vi "Launch.vi"() -> ()   [LabVIEW 2013]
uses:
  Launchcontrol.ctl
panel:
  out "error out":errorcluster
  in  "error in (no error)":errorcluster
  in  "Engaged Angle":i32
  in  "Disengaged Angle":i32
  in  "A":bool
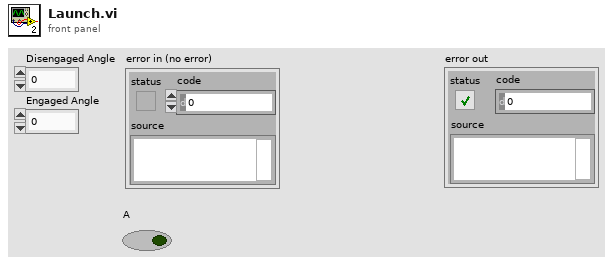
[diagram p1: front panel]
types:
  T1 = typedef "Launchcontrol.ctl" = enum16{"Engaging", "Waiting for Time to Elapse", "Disengaging", "Waiting for Button Press"}
  T2 = typedef "WPI_ServoDeviceRef.ctl" = cluster{"DeviceStatus":errorcluster, "Digital Module":T3, "PWM Channel":T4, "DeadBand":T5}
  T3 = typedef "FPGA_TypedefDigitalModule.ctl" = enum16{"Digital Module 1", "Digital Module 2"}
  T4 = typedef "FPGA_DIOPWMChannel.ctl" = enum8{"PWM 1", "PWM 2", "PWM 3", "PWM 4", "PWM 5", "PWM 6", "PWM 7", "PWM 8", "PWM 9", "PWM 10", "Invalid"}
  T5 = typedef "WPI_PWMDeadband.ctl" = cluster{"Name":string, "maxPositivePwm":i32, "minPositivePwm":i32, "centerPwm":i32, "maxNegativePwm":i32, "minNegativePwm":i32, "angularRange":u16}
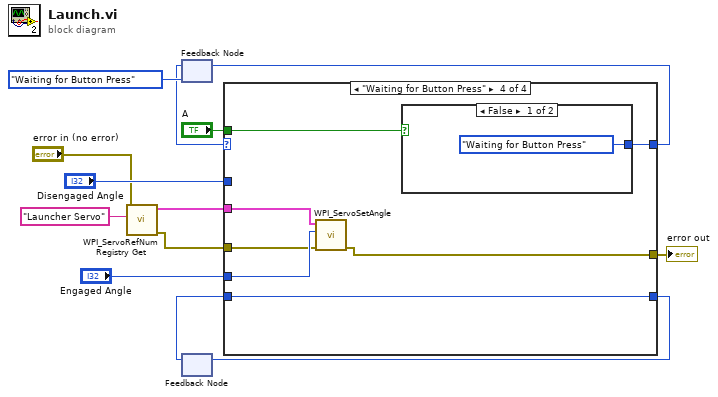
[diagram p0: block diagram]
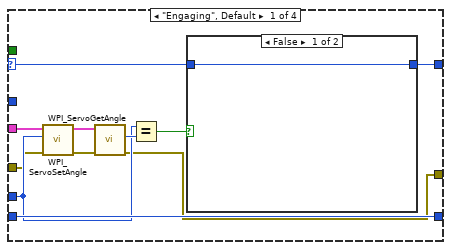
[diagram p2: hidden frame]
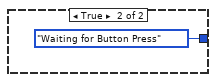
[diagram p3: hidden frame]
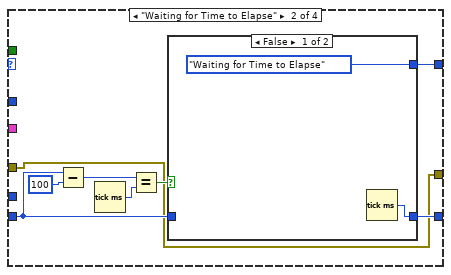
[diagram p4: hidden frame]
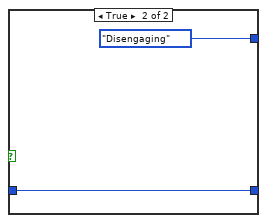
[diagram p5: hidden frame]
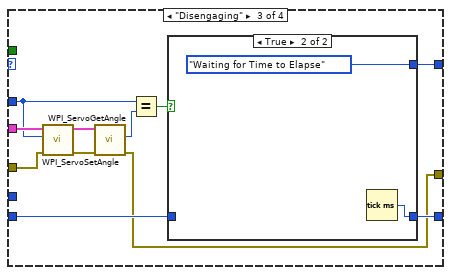
[diagram p6: hidden frame]
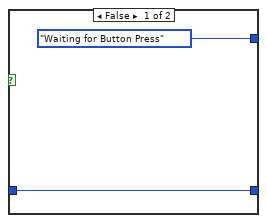
[diagram p7: hidden frame]
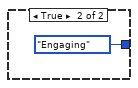
[diagram p8: hidden frame]
diagram:
  n1 = call <vilib>:"WPI_ServoRefNum Registry Get.vi"("error in (no error)"="error in (no error)", "refnum name"="Launcher Servo") -> ("error out"=w3:errorcluster, "ServoDeviceRef"=w8:T2)  [unwired: 8 in]
  n2 = feedback #1(Launchcontrol."Waiting for Button Press") -> (w12:T1)
  n3 = feedback #2() -> (w5:u32)  [unwired: 1 in]
  n4 = case shown="\"Waiting for Button Press\"" w12 {
    selector: w12 -> [w17 _ _ _]
    tunnel: "A" -> [_ _ _ w60]
    tunnel: [w16 w29 w43 w59] -> w10
    tunnel: w8 -> [w19 _ w49 w57]
    tunnel: "Disengaged Angle" -> [_ _ w48 _]
    tunnel: [w24 w30 w42 w58] -> w6
    tunnel: w5 -> [w24 w28 w41 w58]
    tunnel: "Engaged Angle" -> [w18 _ _ w56]
    tunnel: w3 -> [w15 w27 w39 w55]
    tunnel: [w14 w27 w40 w54] -> w1
    frame "Engaging", Default {
      n5 = call <vilib>:"WPI_ServoSetAngle.vi"("error in (no error)"=w15, "Angle"=w18, "ServoDeviceRef"=w19) -> ("error out"=w21:errorcluster, "ServoDeviceRef"=w22:T2)  [unwired: 7 in]
      n6 = call <vilib>:"WPI_ServoGetAngle.vi"("ServoDeviceRef"=w22, "error in (no error)"=w21) -> ("Angle"=w23:u16, "error out"=w14:errorcluster)  [unwired: 6 in, 1 out]
      n7 = Equal?(x=w18, y=w23) -> (x = y?=w20:bool)
      n8 = case shown="False" w20 {
        tunnel: [w25 Launchcontrol."Waiting for Button Press"] -> w16
        tunnel: w17 -> [w25 _]
        frame False {
        }
        frame True {
        }
      }
    }
    frame "Waiting for Time to Elapse" {
      n9 = Subtract(x=w28, y=100) -> (x-y=w32:u32)
      n10 = Tick Count (ms)() -> (millisecond timer value=w34:u32)
      n11 = Equal?(x=w32, y=w34) -> (x = y?=w31:bool)
      n12 = case shown="False" w31 {
        tunnel: [w36 w37] -> w30
        tunnel: [Launchcontrol."Waiting for Time to Elapse" Launchcontrol."Disengaging"] -> w29
        tunnel: w28 -> [_ w37]
        frame False {
          n13 = Tick Count (ms)() -> (millisecond timer value=w36:u32)
        }
        frame True {
        }
      }
    }
    frame "Disengaging" {
      n14 = call <vilib>:"WPI_ServoSetAngle.vi"("error in (no error)"=w39, "Angle"=w48, "ServoDeviceRef"=w49) -> ("error out"=w45:errorcluster, "ServoDeviceRef"=w46:T2)  [unwired: 7 in]
      n15 = call <vilib>:"WPI_ServoGetAngle.vi"("ServoDeviceRef"=w46, "error in (no error)"=w45) -> ("Angle"=w47:u16, "error out"=w40:errorcluster)  [unwired: 6 in, 1 out]
      n16 = Equal?(x=w48, y=w47) -> (x = y?=w44:bool)
      n17 = case shown="True" w44 {
        tunnel: [Launchcontrol."Waiting for Button Press" Launchcontrol."Waiting for Time to Elapse"] -> w43
        tunnel: [w50 w52] -> w42
        tunnel: w41 -> [w50 _]
        frame False {
        }
        frame True {
          n18 = Tick Count (ms)() -> (millisecond timer value=w52:u32)
        }
      }
    }
    frame "Waiting for Button Press" {
      n19 = call <vilib>:"WPI_ServoSetAngle.vi"("error in (no error)"=w55, "Angle"=w56, "ServoDeviceRef"=w57) -> ("error out"=w54:errorcluster)  [unwired: 7 in, 1 out]
      n20 = case shown="False" w60 {
        tunnel: [Launchcontrol."Waiting for Button Press" Launchcontrol."Engaging"] -> w59
        frame False {
        }
        frame True {
        }
      }
    }
  }
  "error out" <- w1
  n21 = feedback-in #1(w10) -> ()
  n22 = feedback-in #2(w6) -> ()
